vi "one button press control subVI.vi"(11 "Boolean in":bool) -> (3 "Boolean out":bool)   [LabVIEW 2017]
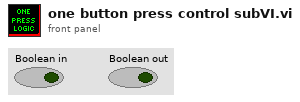
[diagram p1: front panel]
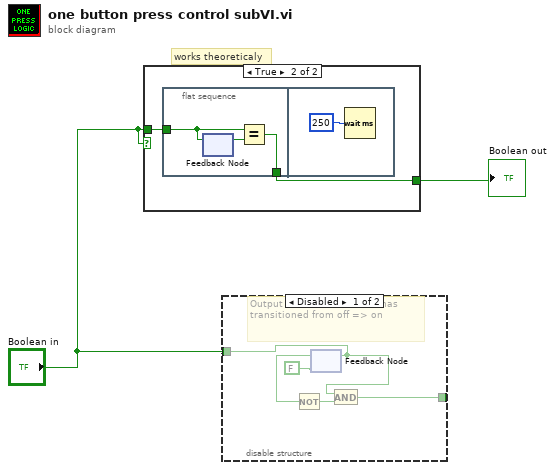
[diagram p0: block diagram]
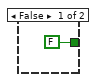
[diagram p3: hidden frame]
diagram:
  # "works theoreticaly"
  n1 = case shown="True" "Boolean in" {
    tunnel: "Boolean in" -> [_ w5]
    tunnel: [FALSE w4] -> w1
    frame False {
    }
    frame True {
      n2 = flat-sequence {
        tunnel: w5 -> [w7]
        tunnel: [w6] -> w4
        frame #0 {
          n3 = feedback #1() -> (w8:bool)  [unwired: 1 in]
          n4 = feedback-in #1(w7) -> ()
          n5 = Equal?(x=w7, y=w8) -> (x = y?=w6:bool)
        }
        frame #1 {
          n6 = Wait (ms)(milliseconds to wait=u32 250 ("millisecond timer value")) -> ()  [unwired: 1 out]
        }
      }
    }
  }
  "Boolean out" <- w1
  n7 = disable-structure shown="Disabled" {
    disable-tunnel: "Boolean in" -> [w11 _]
    disable-tunnel: [w10 _] -> _
    frame Disabled {
      # "Output true when Button 2 has transitioned from off => on"
      n8 = feedback #2(FALSE) -> (w12:bool)
      n9 = Not(x=w12) -> (.not. x?=w13:bool)
      n10 = feedback-in #2(w11) -> ()
      n11 = And(x=w11, y=w13) -> (x .and. y?=w10:bool)
    }
    frame Enabled {
    }
  }
